vi "Profile A Generation v1.vi"() -> ()   [LabVIEW 2018]
uses:
  <vilib>/Utility/file.llb/Write Delimited Spreadsheet (DBL).vi
  <vilib>/addons/Time Series Analysis/Statistical Analysis.llb/TSA Normal Distribution Test (Array).vi
  <vilib>/express/express analysis/Spectral/Block/exnSpectralBlock spectral measurements power poly.vi
  <vilib>/express/express analysis/Spectral/Block/exnSpectralBlock spectral measurements power WFM.vi
  <vilib>/express/express analysis/Spectral/XNode/ExpressSpectralMeasurementsBlockNode.xnode
  <vilib>/addons/_Advanced Signal Processing/NI_AdvSigProcTSA.lvlib
  <vilib>/measure/NI_MABase.lvlib
  <vilib>/Analysis/NI_AALBase.lvlib
panel:
  in  "Frequency":dbl=0.0012505 format="%#_13g"
  in  "Samples":i32=2400
  in  "filter specifications":T1={"lower cutoff freq"=0.1, "higher cutoff freq"=2.0, "order"=5}
  in  "Standard Deviation":dbl=0.0009148153893115104
  in  "exponent 2":dbl=0.8 format="%.2p"
  in  "noise density":dbl=0.47 format="%.2p"
  out "Power Spectrum (Hanning window)":cluster{"f0":dbl, "df":dbl, "magnitude":dbl[]}(graph)
  out "Histogram":cluster{"Axis":dbl[], dbl[]}[](graph)
  out "Data":dbl[][](graph)
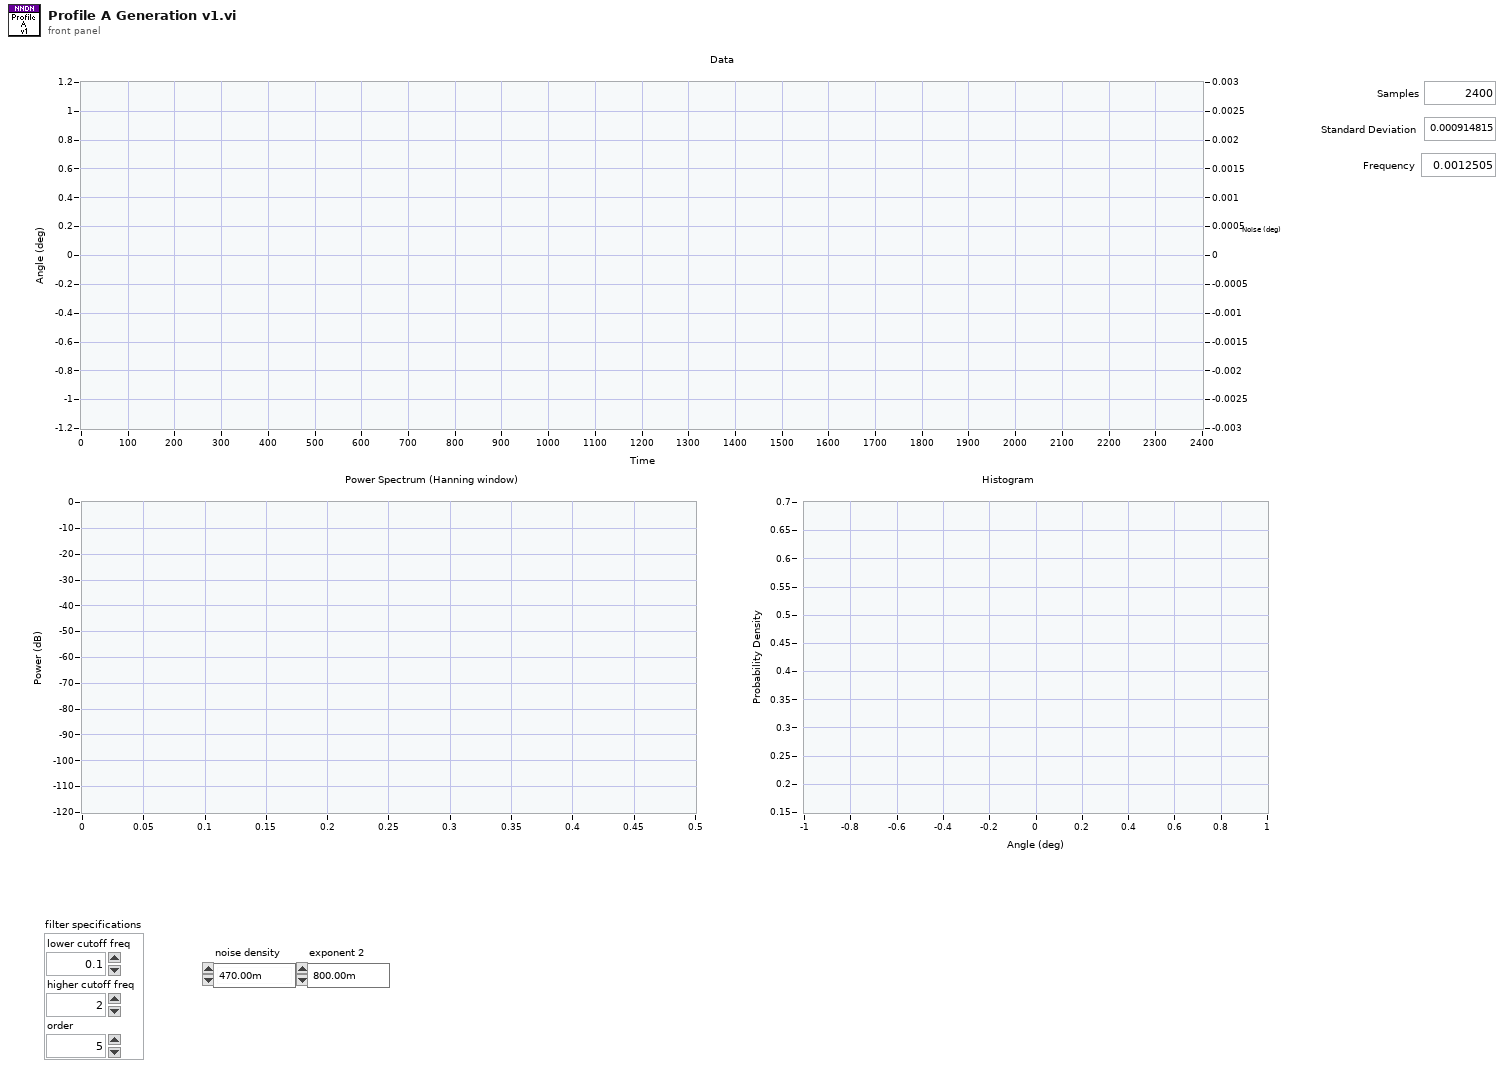
[diagram p1: front panel]
types:
  T1 = cluster{"lower cutoff freq":dbl, "higher cutoff freq":dbl, "order":i32}
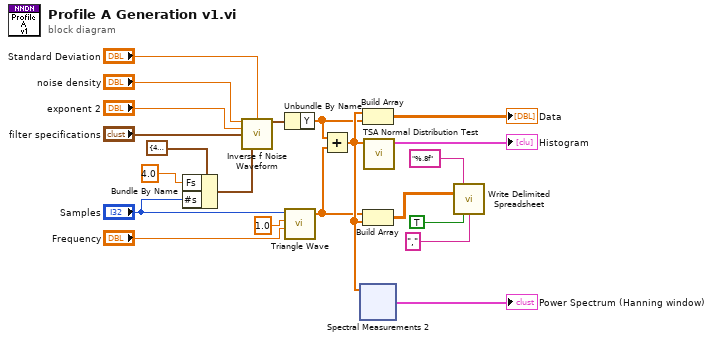
[diagram p0: block diagram]
diagram:
  n1 = Bundle By Name(cluster=cluster{"Fs":dbl, "#s":dbl} {"Fs"=4.0, "#s"=1000.0} ("sampling info"), "Fs"=4.0, "#s"="Samples") -> (w10:cluster{"Fs":dbl, "#s":dbl})
  n2 = call <vilib>:"Inverse f Noise Waveform.vi"("noise density"="noise density", "standard deviation"="Standard Deviation", "exponent"="exponent 2", "filter specifications"="filter specifications", "sampling info"=w10) -> ("signal out"=w12:waveform(dbl))  [unwired: 6 in, 4 out]
  n3 = Unbundle By Name(w12) -> ("Y"=w2:dbl[])
  n4 = call <vilib>:"Triangle Wave.vi"("samples"="Samples", "amplitude"=1.0, "frequency"="Frequency") -> ("triangle wave"=w1:dbl[])  [unwired: 2 in, 2 out]
  n5 = Add(x=w2, y=w1) -> (x+y=w7:dbl[])
  n6 = xnode "Spectral Measurements 2"("Signals"=w7) -> ("Power Spectrum"=→"Power Spectrum (Hanning window)":cluster{"f0":dbl, "df":dbl, "magnitude":dbl[]})  [unwired: 1 in, 1 out]
  n7 = Build Array(w7, w2) -> (→"Data":dbl[][])
  n8 = Build Array(w1, w7) -> (w6:dbl[][])
  n9 = call-poly <vilib>:"TSA Normal Distribution Test.vi"("Xt"=w7) -> ("histogram"=→"Histogram":cluster{"Axis":dbl[], dbl[]}[])  [unwired: 9 in, 1 out]
  n10 = call-poly <vilib>:"Write Delimited Spreadsheet.vi"("format (%.3f)"="%.8f", "2D data"=w6, "transpose? (no:F)"=TRUE, "delimiter (\\t)"="," ("delimiter (\\t)")) -> ()  [unwired: 10 in, 2 out]
